vi "eventos.vi"() -> ()   [LabVIEW 2013]
panel:
  in  "DetenerPrograma":bool
  in  "Llenar":bool
  in  "Llave":bool
  out "Tanques":i32(slide) scale=0.0..1000.0
  # "Tema: Eventos"
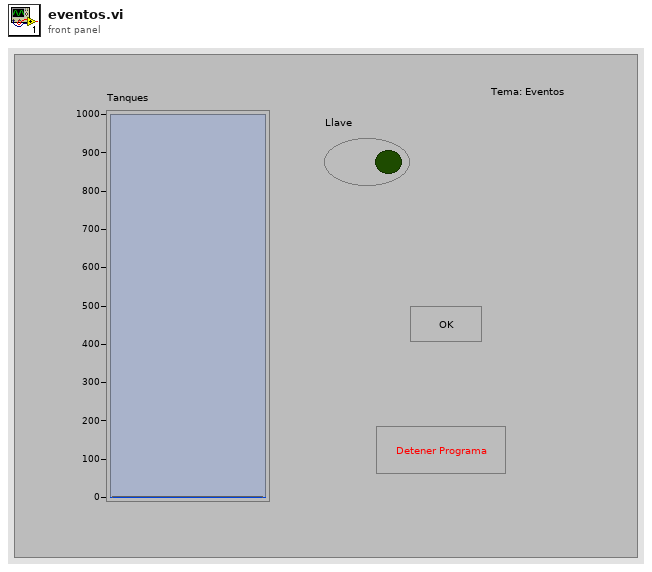
[diagram p1: front panel]
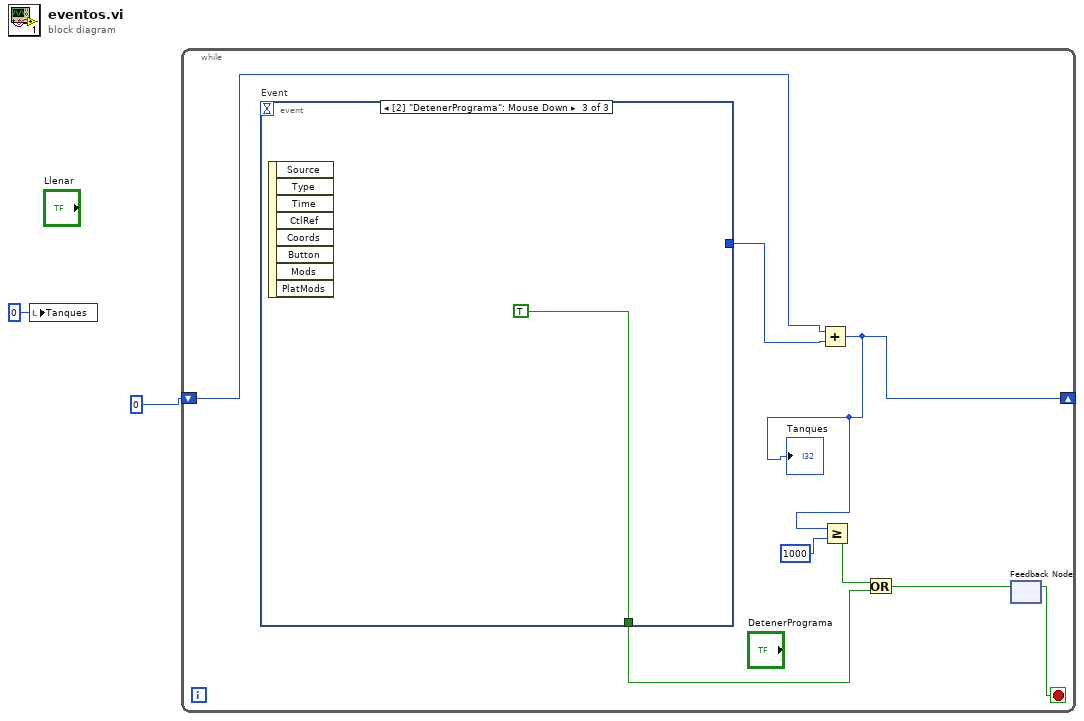
[diagram p0: block diagram]
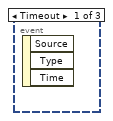
[diagram p2: hidden frame]
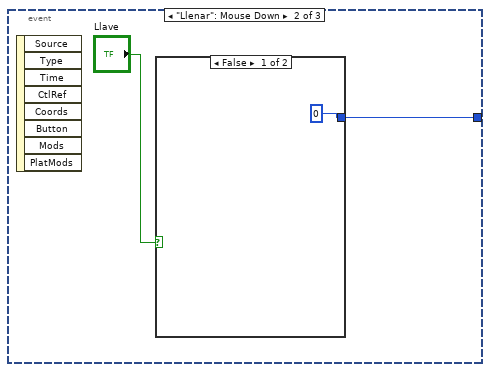
[diagram p3: hidden frame]
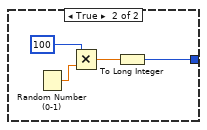
[diagram p4: hidden frame]
diagram:
  n1 = local write "Tanques"(0 ("Tanques")) -> ()
  n2 = while {
    shift-right: [w8] -> _
    shift-left: 0 -> [w10]
    stop <- w4 stop-if-true
    n3 = event "Event" shown="[2] \"DetenerPrograma\": Mouse Down" {
      selector: _ -> [_ _ _]
      dyn-events: _ -> [_ _ _]
      timeout: _ -> [_ _ _]
      tunnel: [_ w11 _] -> w9
      tunnel: [_ _ TRUE] -> w3
      event Timeout {
        n4 = event-data() -> ()  [unwired: 1 in, 3 out]
      }
      event "Llenar": Mouse Down {
        n5 = event-data() -> ()  [unwired: 1 in, 8 out]
        n6 = case shown="False" "Llave" {
          tunnel: [0 w14] -> w11
          frame False {
          }
          frame True {
            n7 = Random Number (0-1)() -> (number: 0 to 1=w16:dbl)
            n8 = Multiply(x=100, y=w16) -> (x*y=w15:dbl)
            n9 = To Long Integer(number=w15) -> (32bit integer=w14:i32)
          }
        }
      }
      event "DetenerPrograma": Mouse Down {
        n10 = event-data() -> ()  [unwired: 1 in, 8 out]
      }
    }
    n11 = Add(x=w10, y=w9) -> (x+y=w8:i32)
    "Tanques" <- w8
    n12 = Greater Or Equal?(x=w8, y=1000) -> (x >= y?=w6:bool)
    n13 = Or(x=w6, y=w3) -> (x .or. y?=w5:bool)
    n14 = feedback-in #1(w5) -> ()
    n15 = feedback #1() -> (w4:bool)  [unwired: 1 in]
  }
